vi "ReadExEventFINAL_new.vi"() -> ()   [LabVIEW 2015]
uses:
  GPS_Driver_Global.vi
panel:
  in  "Path to FITS Header File":path=path "C:/Users/Public/Documents/SI Image SGL II -/Other Parameters.txt"
  out "# Entries After":i16
  in  "# Entries Before":i16
  out "Close Min":u32
  out "Close Maj":u32
  out "Open Min":u32
  out "Open Maj":u32
  out "error out":errorcluster
  in  "error in (no error)":errorcluster
  # "Major UNIX Time:"
  # "Minor UNIX Time:"
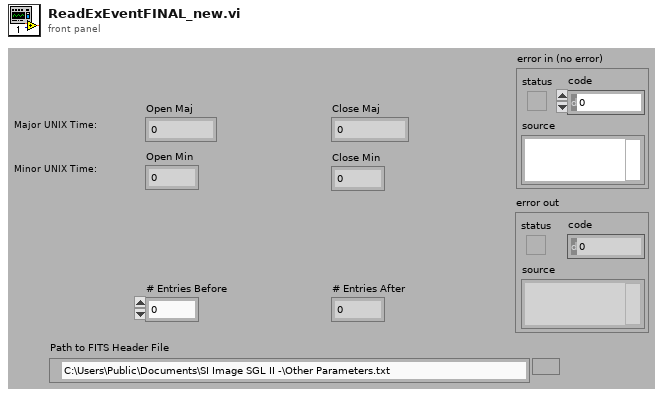
[diagram p1: front panel]
types:
  T1 = cluster{"Close":cluster{"Time":string, "Error":string}, "Open":cluster{"Time":string, "Error":string}, "Date":cluster{"Date":string, "Error":string}}
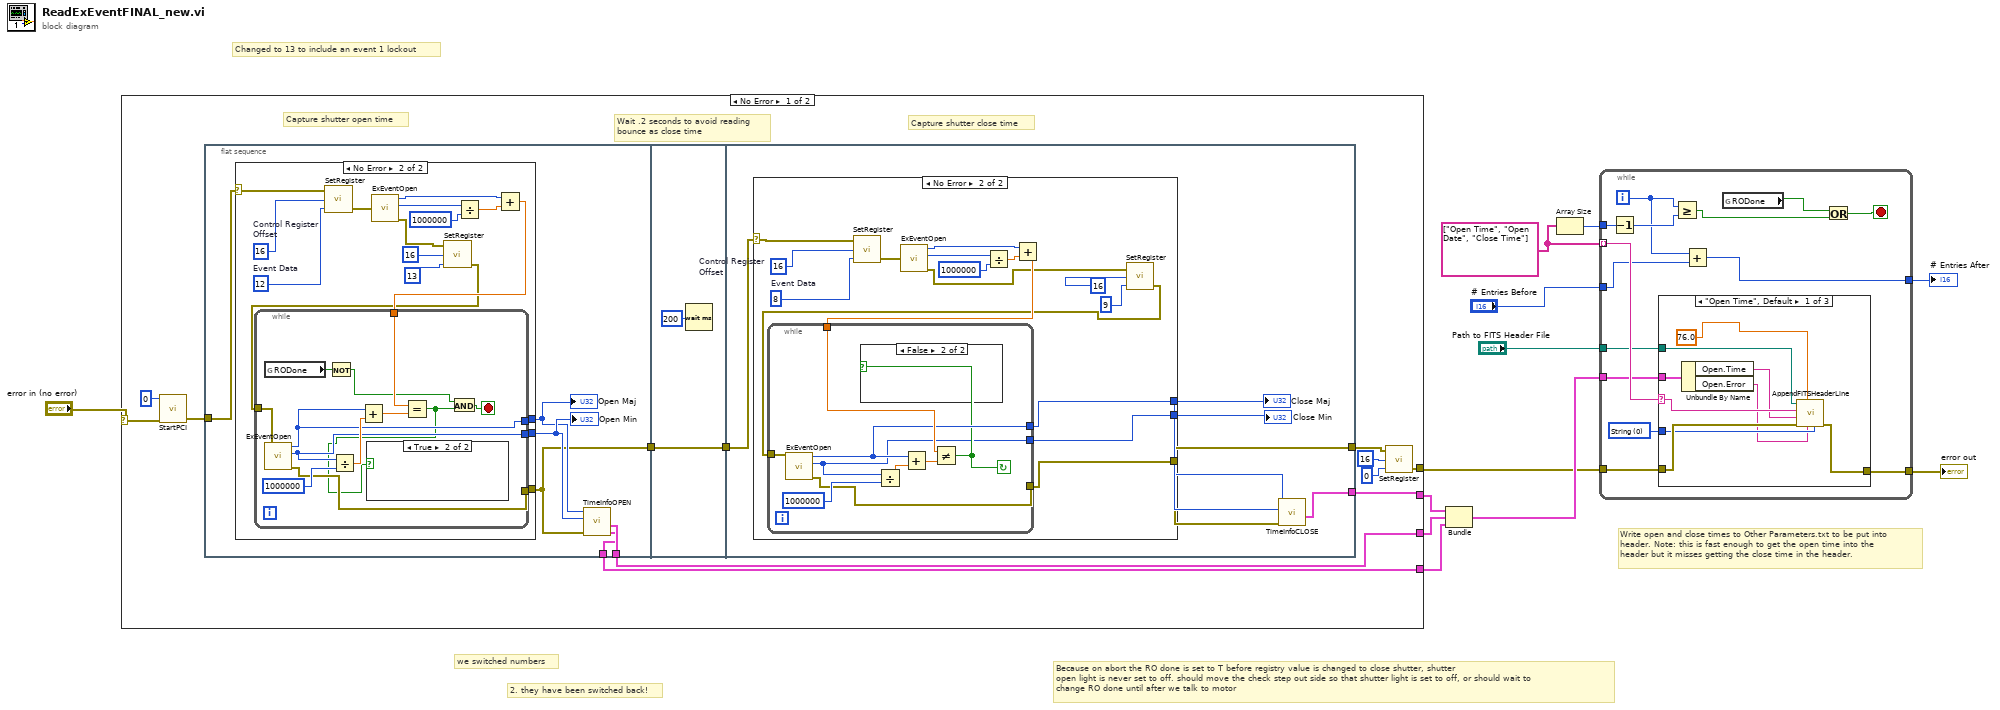
[diagram p0: block diagram]
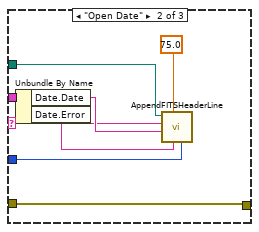
[diagram p2: hidden frame]
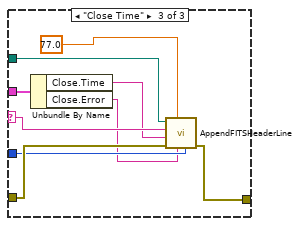
[diagram p3: hidden frame]
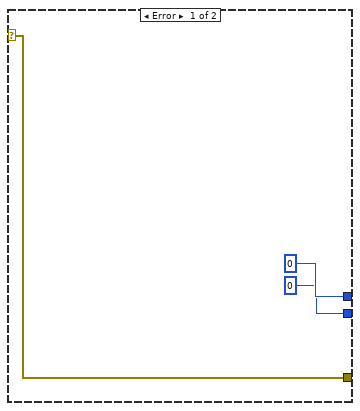
[diagram p4: hidden frame]
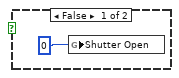
[diagram p5: hidden frame]
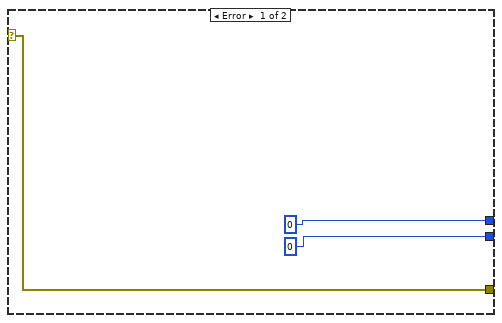
[diagram p6: hidden frame]
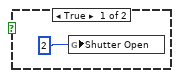
[diagram p7: hidden frame]
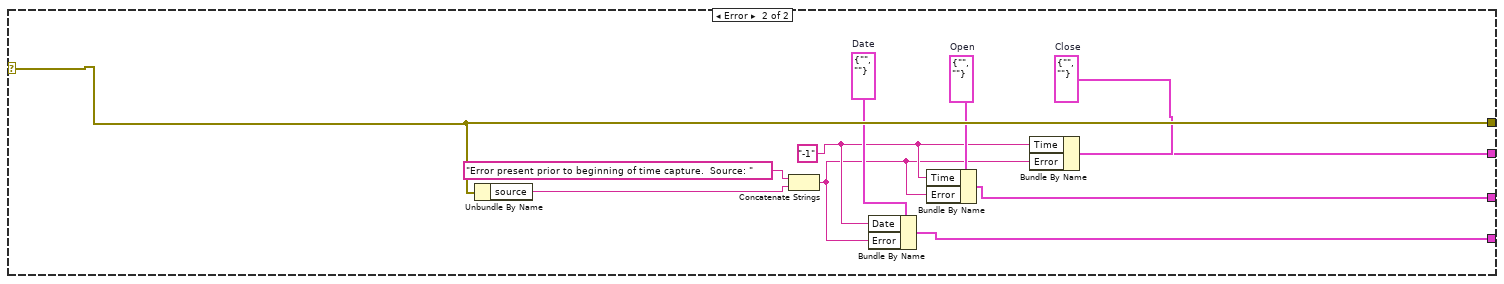
[diagram p8: hidden frame]
diagram:
  w12 = string[] ["Open Time", "Open Date", "Close Time"]
  # "Changed to 13 to include an event 1 lockout"
  # "Because on abort the RO done is set to T before registry value is changed to close shutter, shutter\nopen light is never set to off. should move the check step out side so that shutter light is set to off, or should wait to \nchange RO done until after we talk to motor"
  # "2. they have been switched back!"
  # "we switched numbers"
  # "Write open and close times to Other Parameters.txt to be put into\nheader. Note: this is fast enough to get the open time into the \nheader but it misses getting the close time in the header."
  n1 = case shown="No Error" "error in (no error)" {
    selector: "error in (no error)" -> [w20 w109]
    tunnel: [w21 w109] -> w7
    tunnel: [w18 w102] -> w8
    tunnel: [w17 w105] -> w9
    tunnel: [w14 w103] -> w1
    frame No Error {
      # "Capture shutter close time"
      # "Wait .2 seconds to avoid reading \nbounce as close time"
      # "Capture shutter open time"
      n2 = call "StartPCI.vi"("error in (no error)"=w20, "Device Number"=0) -> ("error out"=w19:errorcluster)  [unwired: 4 in]
      n3 = flat-sequence {
        tunnel: w19 -> [w28]
        tunnel: [w27] -> w18
        tunnel: [w26] -> w16
        tunnel: [w25] -> w14
        tunnel: w16 -> [w63]
        tunnel: [w63] -> w13
        tunnel: [w67] -> w17
        tunnel: [w65] -> w15
        tunnel: w13 -> [w66]
        frame #0 {
          n4 = case shown="No Error" w28 {
            selector: w28 -> [w31 w38]
            tunnel: [0 w47] -> w30
            tunnel: [w31 w46] -> w26
            tunnel: [0 w45] -> w29
            frame Error {
            }
            frame No Error {
              w48 = 12  # Event Data
              w49 = 16  # Control Register Offset
              n5 = call "SetRegister.vi"("Data"=w48, "Offset"=w49, "error in (no error)"=w38) -> ("error out"=w44:errorcluster)  [unwired: 2 in]
              n6 = call "ExEventOpen.vi"("error in (no error)"=w44) -> ("Major Time"=w41:u32, "Minor Time"=w43:u32, "error out"=w35:errorcluster)  [unwired: 1 in]
              n7 = call "SetRegister.vi"("Data"=13 ("Event Data"), "Offset"=16 ("Control Register\nOffset"), "error in (no error)"=w35) -> ("error out"=w34:errorcluster)  [unwired: 2 in]
              n8 = Divide(x=w43, y=1000000) -> (x/y=w40:dbl)
              n9 = Add(x=w41, y=w40) -> (x+y=w39:dbl)
              n10 = while {
                tunnel: w34 -> [w61]
                tunnel: w39 -> [w60]
                tunnel: [w57] -> w46
                tunnel: [w55] -> w45
                tunnel: [w54] -> w47
                stop <- w53 stop-if-true
                n11 = global read "GPS_Driver_Global.vi" "RODone"() -> (w51:bool)
                n12 = call "ExEventOpen.vi"("error in (no error)"=w61) -> ("Major Time"=w55:u32, "Minor Time"=w54:u32, "error out"=w57:errorcluster)  [unwired: 1 in]
                n13 = Not(x=w51) -> (.not. x?=w52:bool)
                n14 = Divide(x=w54, y=1000000) -> (x/y=w59:dbl)
                n15 = Add(x=w55, y=w59) -> (x+y=w56:dbl)
                n16 = Equal?(x=w60, y=w56) -> (x = y?=w50:bool)
                n17 = case shown="True" w50 {
                  frame False {
                    n18 = global write "GPS_Driver_Global.vi" "Shutter Open"(0) -> ()
                  }
                  frame True {
                  }
                }
                n19 = And(x=w52, y=w50) -> (x .and. y?=w53:bool)
              }
            }
          }
          "Open Min" <- w30
          "Open Maj" <- w29
          n20 = call "TimeInfoOPEN.vi"("error in (no error)"=w26, "Minor Time"=w30, "Major Time"=w29) -> ("Date"=w25:cluster{"Date":string, "Error":string}, "Open"=w27:cluster{"Time":string, "Error":string})  [unwired: 6 in]
        }
        frame #1 {
          n21 = Wait (ms)(milliseconds to wait=200) -> ()  [unwired: 1 out]
        }
        frame #2 {
          n22 = case shown="No Error" w66 {
            selector: w66 -> [w70 w78]
            tunnel: [0 w86] -> w69
            tunnel: [w70 w85] -> w65
            tunnel: [0 w84] -> w68
            frame Error {
            }
            frame No Error {
              w87 = 8  # Event Data
              w88 = 16  # Control Register Offset
              n23 = call "SetRegister.vi"("Data"=w87, "Offset"=w88, "error in (no error)"=w78) -> ("error out"=w83:errorcluster)  [unwired: 2 in]
              n24 = call "ExEventOpen.vi"("error in (no error)"=w83) -> ("Major Time"=w80:u32, "Minor Time"=w82:u32, "error out"=w74:errorcluster)  [unwired: 1 in]
              n25 = Divide(x=w82, y=1000000) -> (x/y=w79:dbl)
              n26 = Add(x=w80, y=w79) -> (x+y=w77:dbl)
              n27 = call "SetRegister.vi"("Data"=9 ("Event Data"), "Offset"=16 ("Control Register\nOffset"), "error in (no error)"=w74) -> ("error out"=w73:errorcluster)  [unwired: 2 in]
              n28 = while {
                tunnel: w73 -> [w97]
                tunnel: w77 -> [w96]
                tunnel: [w93] -> w85
                tunnel: [w91] -> w84
                tunnel: [w89] -> w86
                stop <- w90 continue-if-true
                n29 = call "ExEventOpen.vi"("error in (no error)"=w97) -> ("Major Time"=w91:u32, "Minor Time"=w89:u32, "error out"=w93:errorcluster)  [unwired: 1 in]
                n30 = Divide(x=w89, y=1000000) -> (x/y=w95:dbl)
                n31 = Add(x=w91, y=w95) -> (x+y=w92:dbl)
                n32 = Not Equal?(x=w96, y=w92) -> (x != y?=w90:bool)
                n33 = case shown="False" w90 {
                  frame True {
                    n34 = global write "GPS_Driver_Global.vi" "Shutter Open"(2) -> ()
                  }
                  frame False {
                  }
                }
              }
            }
          }
          "Close Maj" <- w68
          "Close Min" <- w69
          n35 = call "TimeInfoCLOSE.vi"("error in (no error)"=w65, "Minor Time"=w69, "Major Time"=w68) -> ("Close"=w67:cluster{"Time":string, "Error":string})  [unwired: 7 in]
        }
      }
      n36 = call "SetRegister.vi"("Data"=0, "Offset"=16, "error in (no error)"=w15) -> ("error out"=w21:errorcluster)  [unwired: 2 in]
    }
    frame Error {
      w101 = cluster{"Date":string, "Error":string} {"Date"="", "Error"=""}  # Date
      w106 = cluster{"Time":string, "Error":string} {"Time"="", "Error"=""}  # Close
      w104 = cluster{"Time":string, "Error":string} {"Time"="", "Error"=""}  # Open
      w100 = "-1"
      n37 = Unbundle By Name(w109) -> ("source"=w107:string)
      n38 = Concatenate Strings("Error present prior to beginning of time capture.  Source: ", w107) -> (w99:string)
      n39 = Bundle By Name(cluster=w101, "Date"=w100, "Error"=w99) -> (w103:cluster{"Date":string, "Error":string})
      n40 = Bundle By Name(cluster=w104, "Time"=w100, "Error"=w99) -> (w102:cluster{"Time":string, "Error":string})
      n41 = Bundle By Name(cluster=w106, "Time"=w100, "Error"=w99) -> (w105:cluster{"Time":string, "Error":string})
    }
  }
  n42 = Bundle("Close"=w9, "Open"=w8, "Date"=w1) -> (w11:T1)  [unwired: 1 in]
  n43 = Array Size(array=w12) -> (size(s)=w5:i32)
  n44 = while {
    tunnel: w7 -> [w123]
    tunnel: w12 -> [w121] mode=indexing
    tunnel: w5 -> [w120]
    tunnel: "# Entries Before" -> [w118]
    tunnel: w11 -> [w116]
    tunnel: "Path to FITS Header File" -> [w115]
    tunnel: [w114] -> w10
    tunnel: [w110] -> w3
    i -> [w117]
    stop <- w112 stop-if-true
    w119 = u16 0 items=["String", "Numeric", "Boolean"]
    n45 = Decrement(x=w120) -> (x-1=w122:i32)
    n46 = case shown="\"Open Time\", Default" w121 {
      selector: w121 -> [w130 w135 w148]
      tunnel: w123 -> [w132 w134 w149]
      tunnel: w119 -> [w131 w139 w147]
      tunnel: w116 -> [w127 w138 w144]
      tunnel: w115 -> [w129 w140 w145]
      tunnel: [w128 w134 w146] -> w114
      frame "Open Time", Default {
        n47 = Unbundle By Name(w127) -> ("Open.Time"=w126:string, "Open.Error"=w125:string)
        n48 = call "AppendFITSHeaderLine.vi"("Entry Type"=w131, "Comment"=w125, "Entry #"=76.0, "error in (no error)"=w132, "Element Value"=w126, "Element Name"=w130, "file path (dialog if empty)"=w129) -> ("error out"=w128:errorcluster)  [unwired: 3 in]
      }
      frame "Open Date" {
        n49 = Unbundle By Name(w138) -> ("Date.Date"=w137:string, "Date.Error"=w136:string)
        n50 = call "AppendFITSHeaderLine.vi"("Entry Type"=w139, "Comment"=w136, "Entry #"=75.0, "Element Value"=w137, "Element Name"=w135, "file path (dialog if empty)"=w140) -> ()  [unwired: 4 in, 1 out]
      }
      frame "Close Time" {
        n51 = Unbundle By Name(w144) -> ("Close.Time"=w143:string, "Close.Error"=w142:string)
        n52 = call "AppendFITSHeaderLine.vi"("Entry Type"=w147, "Comment"=w142, "Entry #"=77.0, "error in (no error)"=w149, "Element Value"=w143, "Element Name"=w148, "file path (dialog if empty)"=w145) -> ("error out"=w146:errorcluster)  [unwired: 3 in]
      }
    }
    n53 = Greater Or Equal?(x=w117, y=w122) -> (x >= y?=w113:bool)
    n54 = Add(x=w117, y=w118) -> (x+y=w110:i32)
    n55 = global read "GPS_Driver_Global.vi" "RODone"() -> (w111:bool)
    n56 = Or(x=w111, y=w113) -> (x .or. y?=w112:bool)
  }
  "error out" <- w10
  "# Entries After" <- w3
